vi "ReadMaxTime.vi"(8 "error in (no error)":errorcluster, 10 "iMaxTimeMilliseconds":u32, 11 "HandleIn":refnum<visa-resource-name>) -> (0 "error out":errorcluster, 3 "HandleOut":refnum<visa-resource-name>)   [LabVIEW 2014, in "SamplerPlugins.lvlib" / "HP3458aDMM.lvclass"]
uses:
  HP3458aDMM.lvclass
  <vilib>/Utility/error.llb/Error Cluster From Error Code.vi
  <vilib>/ErrorRing/Error Ring.xnode
panel:
  out "read buffer 3":string
  out "read buffer 2":string
  out "length":i32
  out "return count":u32
  out "return count 2":u32
  out "read buffer":string
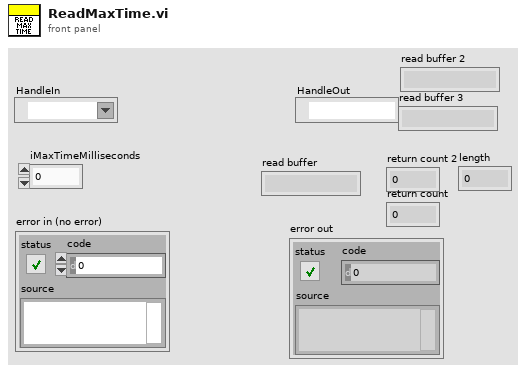
[diagram p1: front panel]
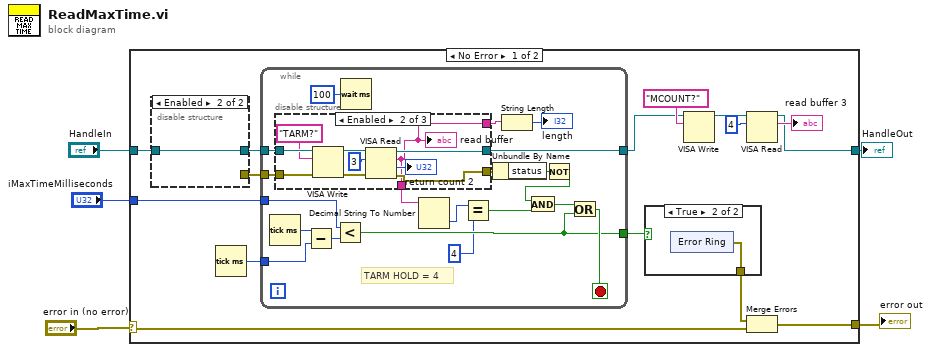
[diagram p0: block diagram]
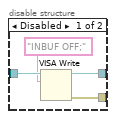
[diagram p2: hidden frame]
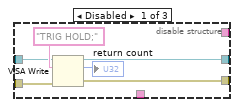
[diagram p3: hidden frame]
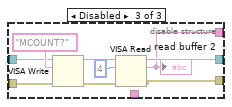
[diagram p4: hidden frame]
diagram:
  n1 = case shown="No Error" "error in (no error)" {
    selector: "error in (no error)" -> [w15 w78]
    tunnel: [w16 w78] -> w4
    tunnel: "HandleIn" -> [w14 w77]
    tunnel: "iMaxTimeMilliseconds" -> [w19 _]
    tunnel: [w6 w77] -> w1
    frame No Error {
      n2 = disable-structure shown="Enabled" {
        disable-tunnel: w14 -> [w24 w25]
        disable-tunnel: [w23 w25] -> w13
        disable-tunnel: [w21 _] -> w12
        frame Disabled {
          n3 = VISA Write(VISA resource name=w24, write buffer="INBUF OFF;") -> (VISA resource name out=w23:refnum<visa-resource-name>, error out=w21:errorcluster)  [unwired: 1 in, 1 out]
        }
        frame Enabled {
        }
      }
      n4 = Tick Count (ms)() -> (millisecond timer value=w20:u32)
      n5 = while {
        tunnel: w13 -> [w44]
        tunnel: [w43] -> w7
        tunnel: w20 -> [w40]
        tunnel: w19 -> [w37]
        tunnel: [w36] -> w18
        tunnel: w12 -> [w35]
        stop <- w39 stop-if-true
        # "TARM HOLD = 4"
        n6 = Tick Count (ms)() -> (millisecond timer value=w41:u32)
        n7 = disable-structure shown="Enabled" {
          disable-tunnel: w44 -> [w50 w61 w69]
          disable-tunnel: [w49 w55 w64] -> w43
          disable-tunnel: w35 -> [w47 w59 w68]
          disable-tunnel: [_ w52 _] -> w29
          disable-tunnel: [_ w52 w62] -> w28
          disable-tunnel: [w48 w54 w63] -> w26
          frame Disabled {
            n8 = VISA Write(VISA resource name=w50, write buffer="TRIG HOLD;", error in (no error)=w47) -> (VISA resource name out=w49:refnum<visa-resource-name>, return count=→"return count":u32, error out=w48:errorcluster)
          }
          frame Enabled {
            n9 = VISA Write(VISA resource name=w61, write buffer="TARM?", error in (no error)=w59) -> (VISA resource name out=w57:refnum<visa-resource-name>, error out=w58:errorcluster)  [unwired: 1 out]
            n10 = VISA Read(VISA resource name=w57, byte count=u32 3, error in (no error)=w58) -> (VISA resource name out=w55:refnum<visa-resource-name>, read buffer=w52:string, return count=→"return count 2":u32, error out=w54:errorcluster)
            "read buffer" <- w52
          }
          frame Disabled {
            n11 = VISA Write(VISA resource name=w69, write buffer="MCOUNT?", error in (no error)=w68) -> (VISA resource name out=w67:refnum<visa-resource-name>, error out=w65:errorcluster)  [unwired: 1 out]
            n12 = VISA Read(VISA resource name=w67, byte count=u32 4, error in (no error)=w65) -> (VISA resource name out=w64:refnum<visa-resource-name>, read buffer=w62:string, error out=w63:errorcluster)  [unwired: 1 out]
            "read buffer 2" <- w62
          }
        }
        n13 = Subtract(x=w41, y=w40) -> (x-y=w38:u32)
        n14 = Less?(x=w37, y=w38) -> (x < y?=w36:bool)
        n15 = Wait (ms)(milliseconds to wait=u32 100) -> ()  [unwired: 1 out]
        n16 = Decimal String To Number(string=w29) -> (number=w30:i32)  [unwired: 2 in, 1 out]
        n17 = Equal?(x=w30, y=u32 4) -> (x = y?=w31:bool)
        n18 = Unbundle By Name(w26) -> ("status"=w42:bool)
        n19 = String Length(string=w28) -> (length=→"length":i32)
        n20 = Not(x=w42) -> (.not. x?=w34:bool)
        n21 = And(x=w34, y=w31) -> (x .and. y?=w33:bool)
        n22 = Or(x=w33, y=w36) -> (x .or. y?=w39:bool)
      }
      n23 = case shown="True" w18 {
        tunnel: [_ w71] -> w17
        frame False {
        }
        frame True {
          n24 = xnode "Error Ring"() -> ("error out"=w71:errorcluster)
        }
      }
      n25 = VISA Write(VISA resource name=w7, write buffer="MCOUNT?") -> (VISA resource name out=w10:refnum<visa-resource-name>)  [unwired: 1 in, 2 out]
      n26 = VISA Read(VISA resource name=w10, byte count=u32 4) -> (VISA resource name out=w6:refnum<visa-resource-name>, read buffer=→"read buffer 3":string)  [unwired: 1 in, 2 out]
      n27 = Merge Errors(w17, w15) -> (w16:errorcluster)
    }
    frame Error {
    }
  }
  "error out" <- w4
  "HandleOut" <- w1
